vi "Read Current Gas Selection.vi"(7 "Unit ID (A)":string="A", 8 "error in":errorcluster, 9 "Gas Selection: Strings and Values":cluster{"Gas Name":string, "Gas number":u16}[](array[cluster]), 10 "Get Gas String":bool, 11 "VISA Session In":refnum<visa-resource-name>="Alicat") -> (0 "error out":errorcluster, 1 "Current Gas Selection (number)":u16, 2 "Current Gas Selection (string)":string, 3 "VISA Session Out":refnum<visa-resource-name>)   [LabVIEW 2015]
doc: "Reads the currently selected gas number and gas name string (if enabled using the boolean). If the gas name string output is enabled, the \"Gas Selection: Strings and Values\" control needs to be wired (this is obtained using the \"Read Gas List\" sub-VI)."
panel:
  # "Strings and names are returned\nfrom the \"Read Gas List\" VI"
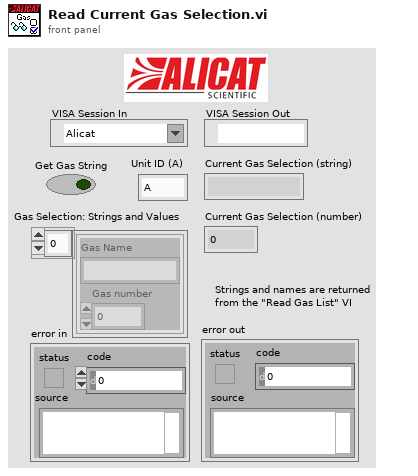
[diagram p1: front panel]
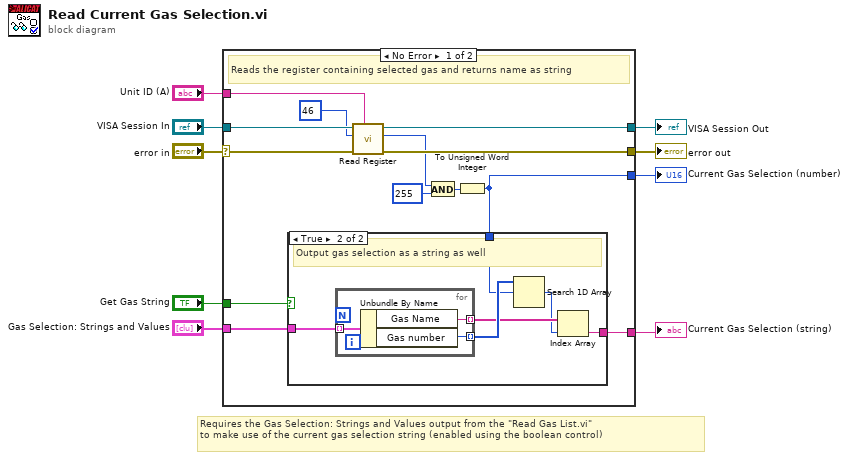
[diagram p0: block diagram]
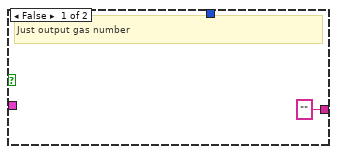
[diagram p2: hidden frame]
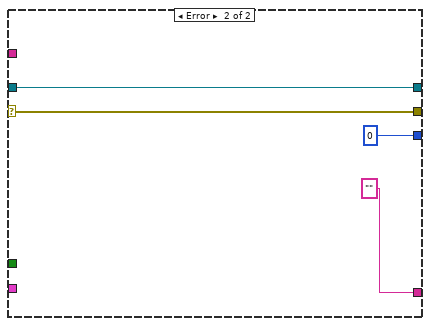
[diagram p3: hidden frame]
diagram:
  # "Requires the Gas Selection: Strings and Values output from the \"Read Gas List.vi\" \nto make use of the current gas selection string (enabled using the boolean control)"
  n1 = case shown="No Error" "error in" {
    selector: "error in" -> [w13 w35]
    tunnel: "Gas Selection: Strings and Values" -> [w21 _]
    tunnel: [w20 "" ("Gas Name")] -> w8
    tunnel: "Unit ID (A)" -> [w19 _]
    tunnel: "VISA Session In" -> [w18 w34]
    tunnel: [w16 w35] -> w5
    tunnel: [w15 w34] -> w4
    tunnel: [w11 u16 0] -> w2
    tunnel: "Get Gas String" -> [w10 _]
    frame No Error {
      # "Reads the register containing selected gas and returns name as string"
      n2 = call "Read Register.vi"("Unit ID (A)"=w19, "error in"=w13, "Register address"=u16 46, "VISA Session In"=w18) -> ("error out"=w16:errorcluster, "Register Value (I32)"=w14:i32, "VISA Session Out"=w15:refnum<visa-resource-name>)  [unwired: 5 in]
      n3 = And(x=w14, y=255) -> (x .and. y?=w12:i32)
      n4 = To Unsigned Word Integer(number=w12) -> (unsigned 16bit integer=w11:u16)
      n5 = case shown="True" w10 {
        tunnel: w21 -> [_ w29]
        tunnel: ["" ("Gas Name") w25] -> w20
        tunnel: w11 -> [_ w24]
        frame False {
          # "Just output gas number"
        }
        frame True {
          # "Output gas selection as a string as well"
          n6 = for {
            tunnel: w29 -> [w32] mode=indexing
            tunnel: [w31] -> w27 mode=indexing
            tunnel: [w30] -> w28 mode=indexing
            n7 = Unbundle By Name(w32) -> ("Gas Name"=w31:string, "Gas number"=w30:u16)
          }
          n8 = Search 1D Array(1D array=w28, element=w24) -> (index of element=w26:i32)  [unwired: 1 in]
          n9 = Index Array(array=w27, index=w26) -> (element=w25:string)
        }
      }
    }
    frame Error {
    }
  }
  "error out" <- w5
  "VISA Session Out" <- w4
  "Current Gas Selection (string)" <- w8
  "Current Gas Selection (number)" <- w2
